vi "Create Sysdef Tree from DB Channel Clusters.vi"(7 "Autocreate Rx timestamp chans?":bool, 8 "error in":errorcluster, 10 "Channels to create":T1, 11 "Device Ptr":u64) -> (0 "error out":errorcluster, 3 "Device Ptr dup":u64)   [LabVIEW 2015, in "AIT 429 System Explorer.lvlib"]
uses:
  AIT 429 System Explorer.lvlib
  Controls/AIT_Channel Array.ctl
  Controls/AIT_Channel.ctl
  Controls/AIT_Label.ctl
  Controls/AIT_Word.ctl
  Controls/ARINCParam.ctl
  Shared/Controls and Global/TransferType.ctl
  <userlib>/ARINC-429/vi/enum/Owl429ChannelSpeed.ctl
  Build Label Properties.vi
  AddParamChannels.vi
  <vilib>/NI Veristand/Custom Device API/NI VeriStand - Add Custom Device Channel.vi
  Shared/Controls and Global/Global.vi
  <vilib>/NI Veristand/Custom Device Tools/Custom Device Utility Library/NI VeriStand - Search for Item by GUID.vi
  <vilib>/NI Veristand/Custom Device API/Custom Device API.lvlib
  Shared/AIT 429 Shared.lvlib
  <vilib>/NI Veristand/Custom Device Tools/Custom Device Utility Library/Custom Device Utility Library.lvlib
  <userlib>/ARINC-429/Owl429.lvlib
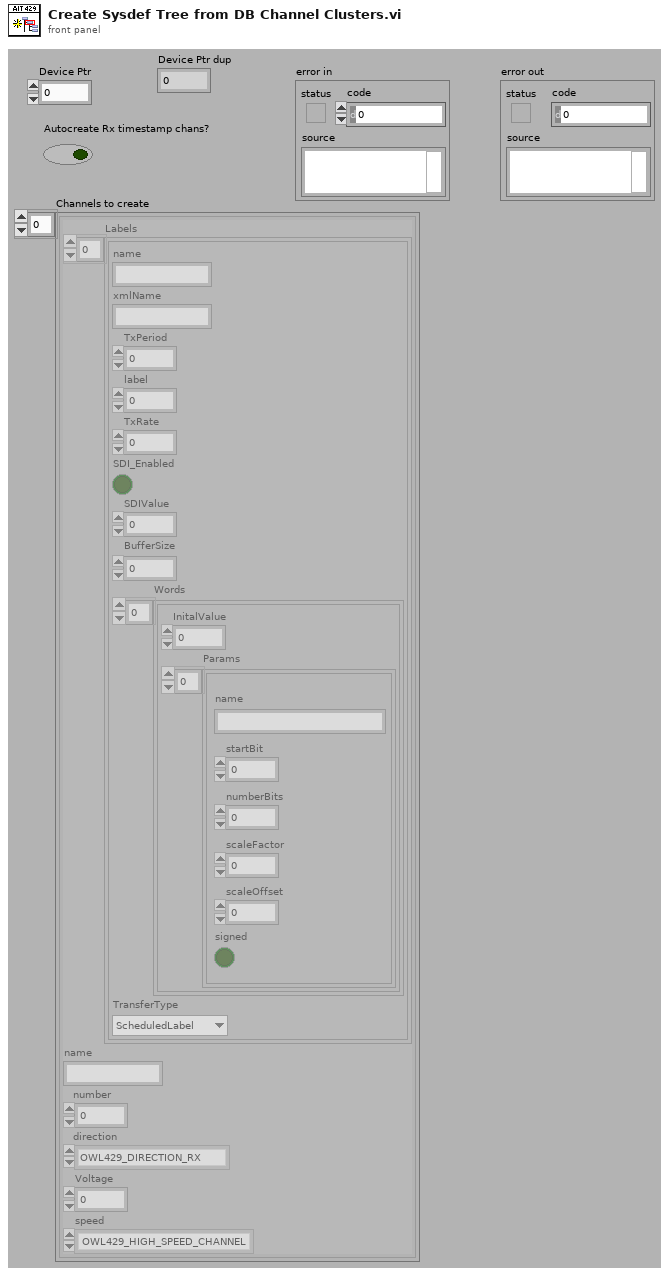
[diagram p1: front panel]
types:
  T1 = typedef "AIT 429 System Explorer.lvlib/AIT_Channel Array.ctl" = T2[]
  T2 = typedef "AIT 429 System Explorer.lvlib/AIT_Channel.ctl" = cluster{"Labels":T3[], "name":string, "number":u8, "direction":enum16{"OWL429_DIRECTION_RX", "OWL429_DIRECTION_TX"}, "Voltage":dbl, "speed":T7}
  T3 = typedef "AIT 429 System Explorer.lvlib/AIT_Label.ctl" = cluster{"name":string, "xmlName":string, "TxPeriod":u32, "label":u32, "TxRate":dbl, "SDI_Enabled":bool, "SDIValue":u8, "BufferSize":u32, "Words":T4[], "TransferType":T6}
  T4 = typedef "AIT 429 System Explorer.lvlib/AIT_Word.ctl" = cluster{"InitalValue":u32, "Params":T5[]}
  T5 = typedef "AIT 429 System Explorer.lvlib/ARINCParam.ctl" = cluster{"name":string, "startBit":i32, "numberBits":i32, "scaleFactor":dbl, "scaleOffset":dbl, "signed":bool}
  T6 = typedef "AIT 429 Shared.lvlib/TransferType.ctl" = enum16{"ScheduledLabel", "Acyclic", "Block", "Strobe"}
  T7 = typedef "Owl429.lvlib/Owl429ChannelSpeed.ctl" = enum16{"OWL429_HIGH_SPEED_CHANNEL", "OWL429_LOW_SPEED_CHANNEL"}
  T8 = enum16{"OWL429_DIRECTION_RX", "OWL429_DIRECTION_TX"}
  T9 = typedef "Custom Device API.lvlib/Custom Device Item Ref.ctl" = u64
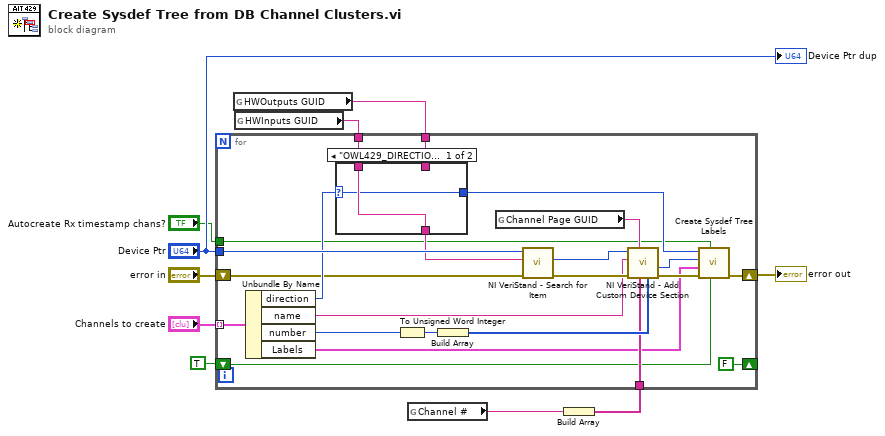
[diagram p0: block diagram]
diagram:
  n1 = global read "Global.vi" "HWOutputs GUID"() -> (w8:string)
  n2 = global read "Global.vi" "HWInputs GUID"() -> (w9:string)
  n3 = global read "Global.vi" "Channel #"() -> (w6:string)
  n4 = Build Array(w6) -> (w7:string[])
  n5 = for {
    tunnel: "Device Ptr" -> [w29]
    shift-right: [w14] -> w4
    shift-left: "error in" -> [w15]
    tunnel: "Channels to create" -> [w30] mode=indexing
    tunnel: w7 -> [w24]
    tunnel: w8 -> [w19]
    tunnel: w9 -> [w20]
    shift-right: [FALSE] -> _
    shift-left: TRUE -> [w13]
    tunnel: "Autocreate Rx timestamp chans?" -> [w11]
    n6 = Unbundle By Name(w30) -> ("direction"=w22:T8, "name"=w26:string, "number"=w25:u8, "Labels"=w18:T3[])
    n7 = case shown="\"OWL429_DIRECTION_RX\"" w22 {
      selector: w22 -> [w34 w36]
      tunnel: [w35 w37] -> w21
      tunnel: w20 -> [w35 _]
      tunnel: w19 -> [_ w37]
      tunnel: [w34 w36] -> w17
      frame "OWL429_DIRECTION_RX" {
      }
      frame "OWL429_DIRECTION_TX" {
      }
    }
    n8 = To Unsigned Word Integer(number=w25) -> (unsigned 16bit integer=w23:u16)
    n9 = Build Array(w23) -> (w32:u16[])
    n10 = global read "Global.vi" "Channel Page GUID"() -> (w31:string)
    n11 = call-poly <vilib>:"NI VeriStand - Search for Item.vi"("error in"=w15, "Item GUID"=w21, "Section Ref in"=w29) -> ("error out"=w27:errorcluster, "Item Ref"=w28:T9)  [unwired: 5 in, 2 out]
    n12 = call <vilib>:"NI VeriStand - Add Custom Device Section.vi"("Property Values"=w32, "Property names"=w24, "GUID (Default Section)"=w31, "error in (no error)"=w27, "Section Name"=w26, "Parent Ref in"=w28) -> ("error out"=w33:errorcluster, "Section Ptr"=w16:T9)  [unwired: 2 in, 2 out]
    n13 = call "Create Sysdef Tree Labels.vi"("first call"=w13, "Autocreate Rx timestamp chans?"=w11, "error in"=w33, "Labels"=w18, "Section Ptr"=w16, "direction"=w17) -> ("error out"=w14:errorcluster)  [unwired: 5 in]
  }
  "error out" <- w4
  "Device Ptr dup" <- "Device Ptr"
